vi "ConstBottomOfChart.vi"() -> (3 "bottom of rectagle":i16)   [LabVIEW 2014]
panel:
  # "położenie prostokąta wykorzystywanaego na wykresie zaczyna się w pkt 150 tzn początek wykresu"
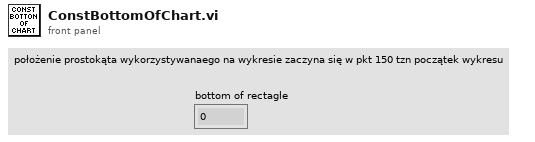
[diagram p1: front panel]
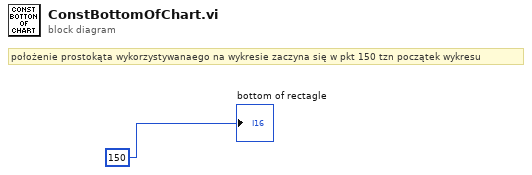
[diagram p0: block diagram]
diagram:
  # "położenie prostokąta wykorzystywanaego na wykresie zaczyna się w pkt 150 tzn początek wykresu"
  "bottom of rectagle" <- i16 150
